vi "set led intensities.vi"(0 "Setpoints":T1(array[cluster]), 2 "Abort Ref":refnum<vi>, 11 "error in":errorcluster) -> (15 "error out":errorcluster)   [LabVIEW 2018]
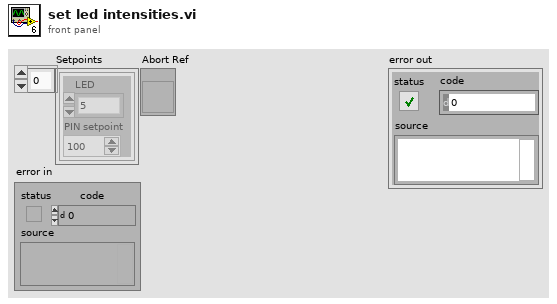
[diagram p1: front panel]
types:
  T1 = cluster{"LED":enum16{"5", "6", "10", "13", "24", "28"}, "PIN setpoint":i32}[]
  T2 = typedef "WindowHandle" = refnum<k1>
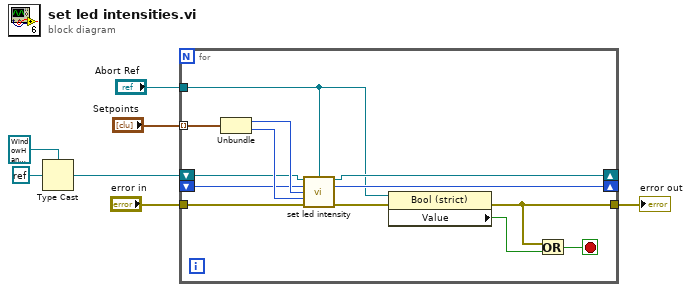
[diagram p0: block diagram]
diagram:
  n1 = Type Cast(type=T2 refnum ("WindowHandle out"), x=refnum<k0> refnum) -> (*(type *) &x=w3:T2)
  n2 = for {
    tunnel: "Setpoints" -> [w20] mode=indexing
    tunnel: "error in" -> [w17]
    tunnel: "Abort Ref" -> [w11]
    shift-right: [w15] -> _
    shift-left: w3 -> [w12]
    shift-right: [w14] -> _
    shift-left: _ -> [w13]
    tunnel: [w8] -> w1
    stop <- w16 stop-if-true
    n3 = Unbundle(w20) -> ("LED"=w19:enum16{"5", "6", "10", "13", "24", "28"}, "PIN setpoint"=w18:i32)
    n4 = call "set led intensity.vi"("WindowHandle in"=w12, "Abort Ref"=w11, "HWND in"=w13, "LED"=w19, "PIN setpoint"=w18, "error in"=w17) -> ("WindowHandle out"=w15:T2, "HWND out"=w14:u32, "error out"=w10:errorcluster)  [unwired: 7 in]
    n5 = property on="Property Node" class="Bool (strict)"(reference=w11, error in=w10) -> (error out=w8:errorcluster, "Value"=w9:bool)  [unwired: 1 out]
    n6 = Or(x=w8, y=w9) -> (x .or. y?=w16:bool)
  }
  "error out" <- w1
